vi "MDF4 Create File.vi"(6 "path in":path, 7 "Error In":errorcluster, 9 "History":T1={"History"="my History", "ID"="LabVIEW Logger", "Vendor"="National Instruments", "Version"="1.0"}, 10 "MDF4 File Path":path) -> (0 "Error Out":errorcluster, 3 "MDF4 File Reference out":i64)   [LabVIEW 2019, in "MD4Logger Engine.lvlib"]
uses:
  MD4Logger Engine.lvlib
  <vilib>/Utility/error.llb/Error Cluster From Error Code.vi
  <vilib>/ErrorRing/Error Ring.xnode
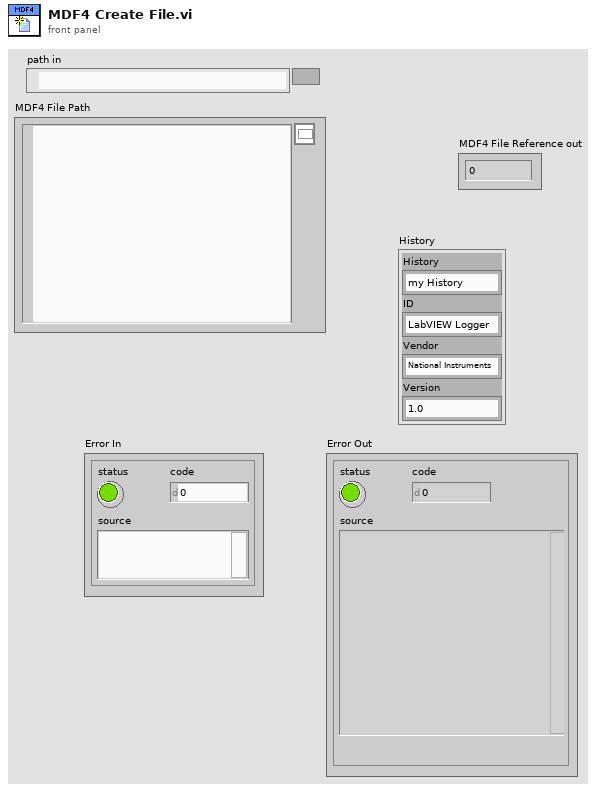
[diagram p1: front panel]
types:
  T1 = cluster{"History":string, "ID":string, "Vendor":string, "Version":string}
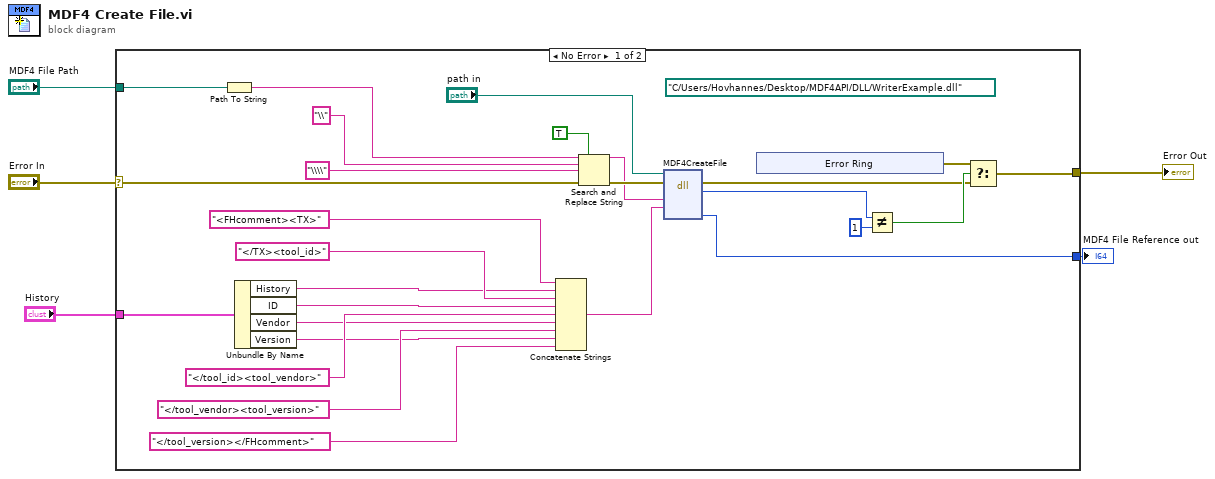
[diagram p0: block diagram]
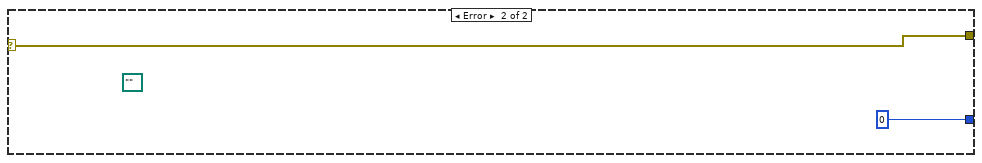
[diagram p2: hidden frame]
diagram:
  n1 = case shown="No Error" "Error In" {
    selector: "Error In" -> [w13 w39]
    tunnel: [w19 w39] -> w4
    tunnel: "MDF4 File Path" -> [w32 _]
    tunnel: [w31 i64 0 ("pFileWriter")] -> w2
    tunnel: "History" -> [w24 _]
    frame No Error {
      (unwired) path "C:/Users/Hovhannes/Desktop/MDF4API/DLL/WriterExample.dll" ("path in")
      n2 = Path To String(path=w32) -> (string=w16:string)
      n3 = Unbundle By Name(w24) -> ("History"=w23:string, "ID"=w22:string, "Vendor"=w21:string, "Version"=w20:string)
      n4 = Concatenate Strings("<FHcomment><TX>", w23, "</TX><tool_id>", w22, "</tool_id><tool_vendor>", w21, "</tool_vendor><tool_version>", w20, "</tool_version></FHcomment>") -> (w27:string)
      n5 = Search and Replace String(replace all?=TRUE ("replace all? (F)"), input string=w16, search string="\\", replace string="\\\\", error in=w13) -> (result string=w6:string, error out=w12:errorcluster)  [unwired: 3 in, 2 out]
      n6 = dll-call lib="C:/Users/Hovhannes/Desktop/MD4Logger/Source/Engine/DLL/WriterExample.dll" fn="MDF4CreateFile"(path in="path in", error in=w12, "path"=w6, "file_history"=w27) -> (error out=w9:errorcluster, "return type"=w8:i32, "m4"=w31:i64)  [unwired: 4 in, 1 out]
      n7 = xnode "Error Ring"() -> ("error out"=w18:errorcluster)
      n8 = Not Equal?(x=w8, y=1) -> (x != y?=w11:bool)
      n9 = Select(t=w18, s=w11, f=w9) -> (s? t:f=w19:errorcluster)
    }
    frame Error {
      (unwired) path "" ("path out")
    }
  }
  "MDF4 File Reference out" <- w2
  "Error Out" <- w4
